vi "Recreate Client.vi"(8 "error in":errorcluster, 11 "grpc client id in":T1) -> (0 "error out":errorcluster, 3 "grpc client id out":T1)   [LabVIEW 2020, in "MeasurementLink Session Management V1.lvlib" / "Session Reservation.lvclass"]
uses:
  Session Reservation.lvclass
  <vilib>/gRPC/LabVIEW gRPC Library/Shared/grpcId.ctl
  MeasurementLink Session Management Client/MeasurementLink Session Management Client.lvlib
  <vilib>/gRPC/LabVIEW gRPC Library/grpc-lvsupport-release.lvlib
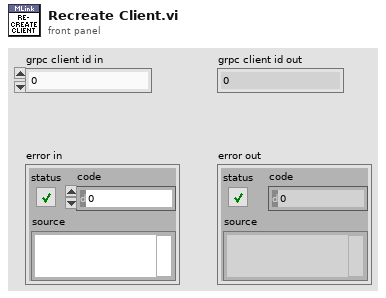
[diagram p1: front panel]
types:
  T1 = typedef "grpc-lvsupport-release.lvlib/grpcId.ctl" = u64
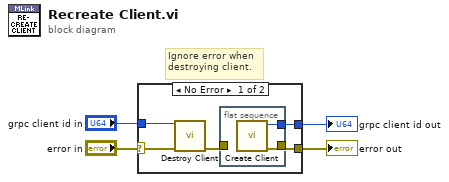
[diagram p0: block diagram]
diagram:
  # "Ignore error when\ndestroying client."
  n1 = case shown="No Error" "error in" {
    selector: "error in" -> [w8 w12]
    tunnel: [w7 w12] -> w3
    tunnel: [w6 _] -> w2
    tunnel: "grpc client id in" -> [w5 _]
    frame No Error {
      n2 = call "Destroy Client.vi"("error in"=w8, "gRPC ID"=w5) -> ("error out"=w9:errorcluster)  [unwired: 9 in]
      n3 = flat-sequence {
        tunnel: w9 -> [_]
        tunnel: [w11] -> w7
        tunnel: [w10] -> w6
        frame #0 {
          n4 = call "Create Client.vi"() -> ("error out"=w11:errorcluster, "grpc client id"=w10:T1)  [unwired: 10 in]
        }
      }
    }
    frame Error {
    }
  }
  "error out" <- w3
  "grpc client id out" <- w2
